vi "swabian_check_sync.vi"(8 "error in (no error)":errorcluster, 10 "Reference\nChannel":T1, 11 "swabian_local_data_IN":T2={"events"={"update_status"=refnum, "update_chart"=refnum, "update_xy"=refnum, "send_channel_data"=refnum}, "stop_q"=refnum, "tagger_reference"=refnum, "connect_button"=refnum, "counter_reference"=refnum, "tagger_stream_reference"=refnum, "log_reference"=refnum, "current_log_offset"=0, "tt20_buffer_q"=refnum, "stream_to_file_button"=refnum, "num_records"=0, "connected?"=FALSE, "plots"=refnum, "histogram_bin_edges"=[], "histogrammer"=refnum, "plot_lifetimes"=refnum, "xy_graph"=refnum, "Reference\nChannel"=enum."ch0", "trigger_channels"=[], "filter_channels"=[], "active_channels"=[], "acq_mode"=0, "Reference\nChannel"=enum."ch0", "acq_time"=0, "leftovers"={"leftover_stamps"=[], "leftover_channels"=[], "any?"=FALSE}, "sync_period_ps"=0, "raw_stream_path"=path "", "Leftovers"={"missing_sync_data"=[], "missing_events"=0}, "first_batch"=0, "first_sync_stamp"=0, "lifetime_settings"={"Plot Lifetimes"=FALSE, "start_time"=0.0, "stop_time"=0.0, "n_bins"=0}, "Histogram_bins"=[], "last_processed_data"=[], "histogram_data"=[]}) -> (0 "error out":errorcluster, 2 "sync_rate_hz":dbl, 3 "swabian_local_data":T2={"events"={"update_status"=refnum, "update_chart"=refnum, "update_xy"=refnum, "send_channel_data"=refnum}, "stop_q"=refnum, "tagger_reference"=refnum, "connect_button"=refnum, "counter_reference"=refnum, "tagger_stream_reference"=refnum, "log_reference"=refnum, "current_log_offset"=0, "tt20_buffer_q"=refnum, "stream_to_file_button"=refnum, "num_records"=0, "connected?"=FALSE, "plots"=refnum, "histogram_bin_edges"=[], "histogrammer"=refnum, "plot_lifetimes"=refnum, "xy_graph"=refnum, "Reference\nChannel"=enum."ch0", "trigger_channels"=[], "filter_channels"=[], "active_channels"=[], "acq_mode"=0, "Reference\nChannel"=enum."ch0", "acq_time"=0, "leftovers"={"leftover_stamps"=[], "leftover_channels"=[], "any?"=FALSE}, "sync_period_ps"=0, "raw_stream_path"=path "", "Leftovers"={"missing_sync_data"=[], "missing_events"=0}, "first_batch"=0, "first_sync_stamp"=0, "lifetime_settings"={"Plot Lifetimes"=FALSE, "start_time"=0.0, "stop_time"=0.0, "n_bins"=0}, "Histogram_bins"=[], "last_processed_data"=[], "histogram_data"=[]})   [LabVIEW 2018]
uses:
  swabian_local_data_tdef.ctl
  swabian_events_tdef.ctl
  update_chart_tdef.ctl
  channel_data_tdef.ctl
  C:/Users/bspoka/Documents/swabian_LV/lib/TTCSharp32.dll
  lib/TTCSharp32.dll
  swabian_buffer_tdef.ctl
  reference_checkbox_tdef.ctl
  leftovers_struct.ctl
  lifetime_settings.ctl
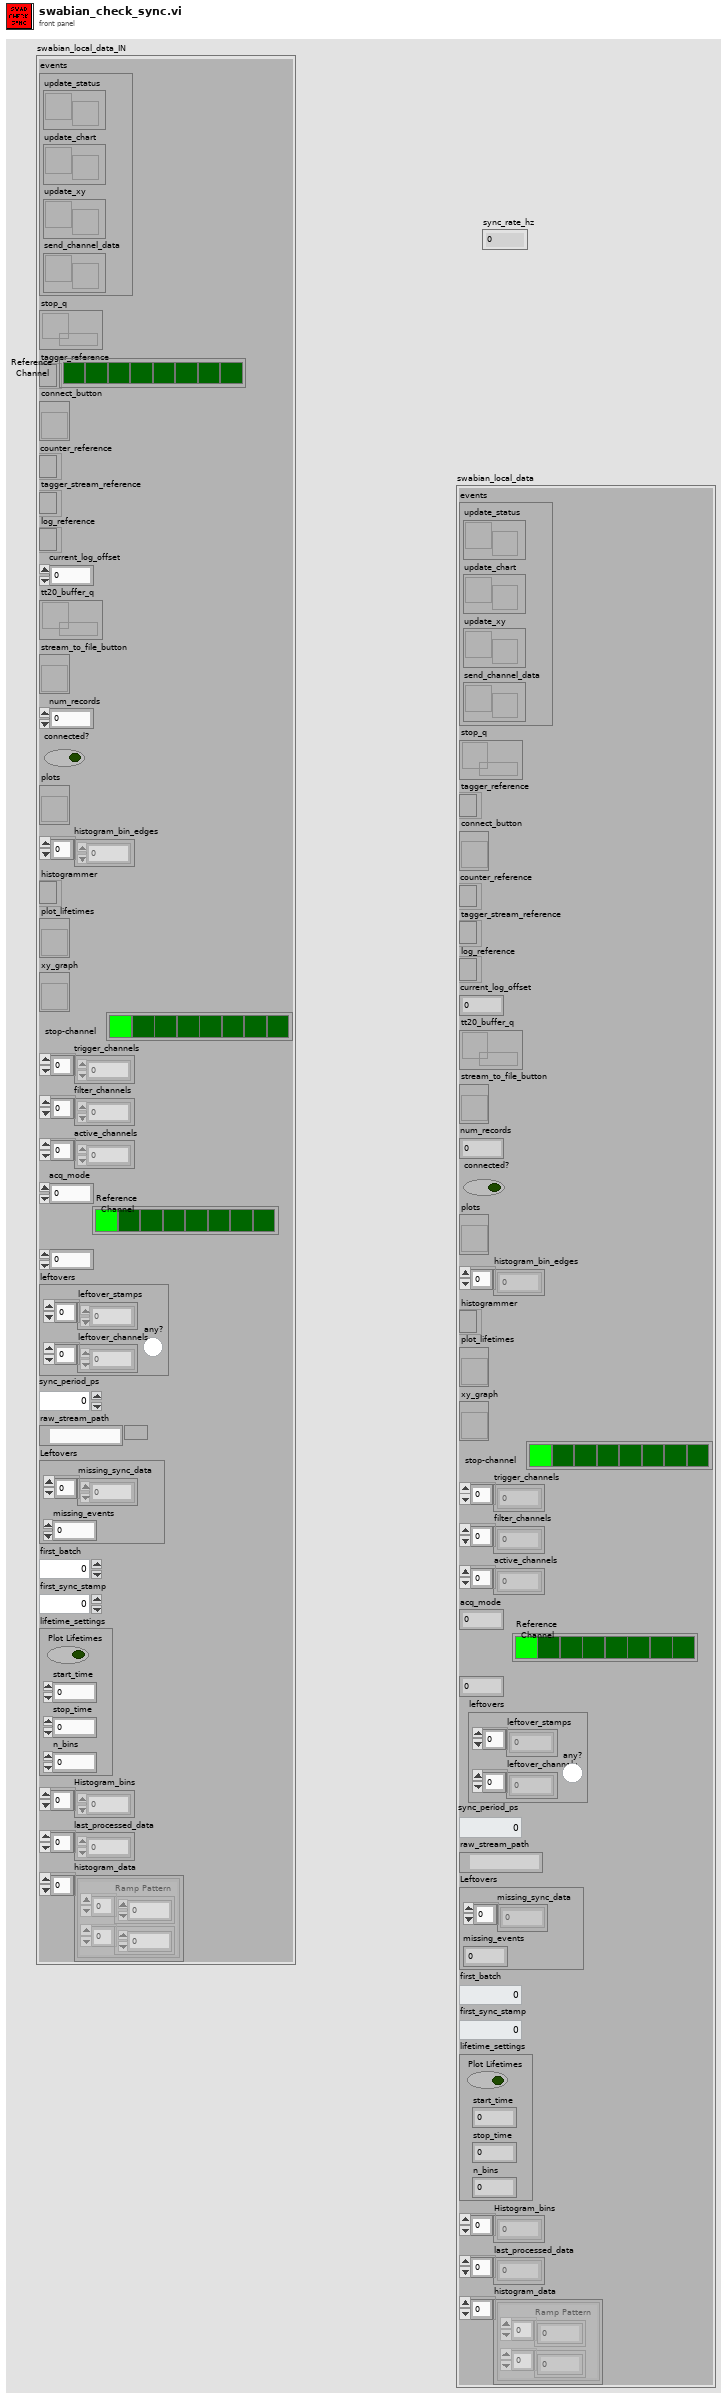
[diagram p1: front panel]
types:
  T1 = typedef "reference_checkbox_tdef.ctl" = enum32{"No Selection", "ch0", "ch1", "ch2", "ch3", "ch4", "ch5", "ch6", "ch7"}
  T2 = typedef "swabian_local_data_tdef.ctl" = cluster{"events":T3, "stop_q":refnum<queue>, "tagger_reference":refnum<k24>, "connect_button":refnum<vi>, "counter_reference":refnum<k24>, "tagger_stream_reference":refnum<k24>, "log_reference":refnum<file>, "current_log_offset":i64, "tt20_buffer_q":refnum<queue>, "stream_to_file_button":refnum<vi>, "num_records":u64, "connected?":bool, "plots":refnum<vi>, "histogram_bin_edges":i64[], "histogrammer":refnum<k24>, "plot_lifetimes":refnum<vi>, "xy_graph":refnum<vi>, "Reference\nChannel":T1, "trigger_channels":i32[], "filter_channels":i32[], "active_channels":i32[], "acq_mode":i32, "Reference\nChannel":T1, "acq_time":i64, "leftovers":T4, "sync_period_ps":i64, "raw_stream_path":path, "Leftovers":cluster{"missing_sync_data":u64[], "missing_events":i32}, "first_batch":i32, "first_sync_stamp":u64, "lifetime_settings":T5, "Histogram_bins":dbl[], "last_processed_data":u64[], "histogram_data":cluster{"Ramp Pattern":dbl[], dbl[]}[]}
  T3 = typedef "swabian_events_tdef.ctl" = cluster{"update_status":refnum<user-event>, "update_chart":refnum<user-event>, "update_xy":refnum<user-event>, "send_channel_data":refnum<user-event>}
  T4 = typedef "leftovers_struct.ctl" = cluster{"leftover_stamps":i64[], "leftover_channels":i32[], "any?":bool}
  T5 = typedef "lifetime_settings.ctl" = cluster{"Plot Lifetimes":bool, "start_time":dbl, "stop_time":dbl, "n_bins":i32}
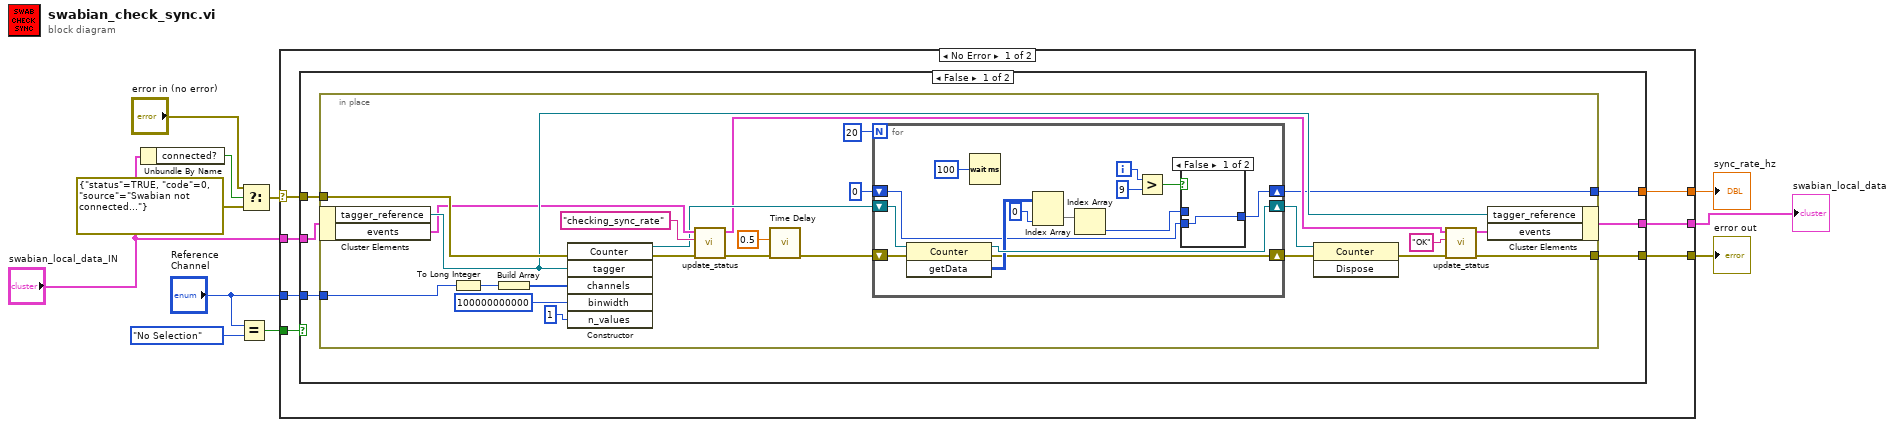
[diagram p0: block diagram]
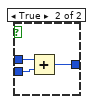
[diagram p2: hidden frame]
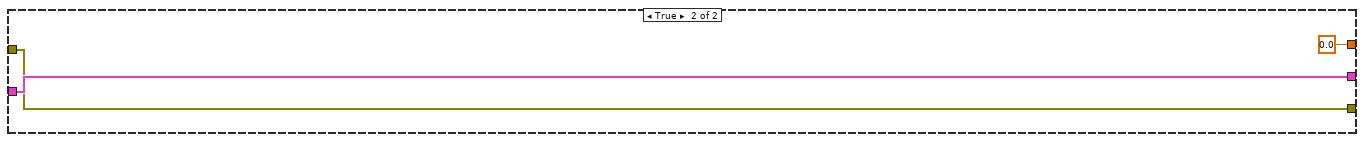
[diagram p3: hidden frame]
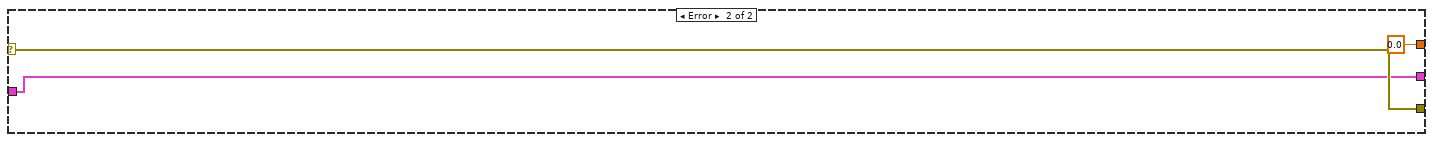
[diagram p4: hidden frame]
diagram:
  n1 = Unbundle By Name("swabian_local_data_IN") -> ("connected?"=w9:bool)
  n2 = Equal?(x="Reference\nChannel", y=reference_checkbox_tdef."No Selection") -> (x = y?=w3:bool)
  n3 = Select(t="error in (no error)", s=w9, f=errorcluster {"status"=TRUE, "code"=0, "source"="Swabian not connected..."}) -> (s? t:f=w5:errorcluster)
  n4 = case shown="No Error" w5 {
    selector: w5 -> [w17 w72]
    tunnel: "swabian_local_data_IN" -> [w18 w71]
    tunnel: [w16 w72] -> w11
    tunnel: [w15 w71] -> w10
    tunnel: w3 -> [w14 _]
    tunnel: "Reference\nChannel" -> [w13 _]
    tunnel: [w12 0.0] -> w1
    frame No Error {
      n5 = case shown="False" w14 {
        tunnel: w18 -> [w24 w69]
        tunnel: w17 -> [w23 w68]
        tunnel: [w22 w68] -> w16
        tunnel: [w21 w69] -> w15
        tunnel: w13 -> [w20 _]
        tunnel: [w19 0.0] -> w12
        frame False {
          n6 = in-place {
            in-place-border: w23 -> [w46]
            in-place-border: [w29] -> w22
            in-place-border: w20 -> [w40]
            in-place-border: [w25] -> w19
            n7 = in-place-cluster #1(w24) -> ("tagger_reference"=w45:refnum<k24>, "events"=w43:T3)
            n8 = To Long Integer(number=w40) -> (32bit integer=w39:i32)
            n9 = Build Array(w39) -> (w41:i32[])
            n10 = constructor class="Counter"(error in=w46, "tagger"=w45, "channels"=w41, "binwidth"=i64 100000000000, "n_values"=1) -> (reference out=w37:refnum<k24>, error out=w44:errorcluster)  [unwired: 2 in, 5 out]
            n11 = call "update_status.vi"("error in (no error)"=w44, "status"="checking_sync_rate", "events"=w43) -> ("error out"=w35:errorcluster, "events_out"=w28:T3)  [unwired: 7 in]
            n12 = call "Time Delay"("error in (no error)"=w35, "Delay Time (s)"=0.5) -> ("error out"=w34:errorcluster)  [unwired: 9 in]
            n13 = for {
              N: 20 -> [_]
              shift-right: [w52] -> w31
              shift-left: w34 -> [w60]
              shift-right: [w59] -> w32
              shift-left: w37 -> [w61]
              shift-right: [w55] -> w25
              shift-left: 0 ("element") -> [w53]
              i -> [w51]
              n14 = invoke class="Counter" method="getData"(reference=w61, error in=w60) -> (reference out=w59:refnum<k24>, error out=w52:errorcluster, "getData"=w58:i32[][])  [unwired: 1 in]
              n15 = Wait (ms)(milliseconds to wait=u32 100) -> ()  [unwired: 1 out]
              n16 = Index Array(array=w58, index (col)=0 ("index (row)")) -> (element=w56:i32[])  [unwired: 1 in]
              n17 = Index Array(array=w56) -> (element=w54:i32)  [unwired: 1 in]
              n18 = Greater?(x=w51, y=9) -> (0:w49:bool)
              n19 = case shown="False" w49 {
                tunnel: [w63 w66] -> w55
                tunnel: w54 -> [_ w65]
                tunnel: w53 -> [w63 w64]
                frame False {
                }
                frame True {
                  n20 = Add(x=w65, y=w64) -> (x+y=w66:i32)
                }
              }
            }
            n21 = invoke class="Counter" method="Dispose"(reference=w32, error in=w31) -> (error out=w30:errorcluster)  [unwired: 1 in, 2 out]
            n22 = call "update_status.vi"("error in (no error)"=w30, "status"="OK", "events"=w28) -> ("error out"=w29:errorcluster, "events_out"=w27:T3)  [unwired: 7 in]
            n23 = in-place-cluster #1("tagger_reference"=w45, "events"=w27) -> (w21:T2)
          }
        }
        frame True {
        }
      }
    }
    frame Error {
    }
  }
  "error out" <- w11
  "swabian_local_data" <- w10
  "sync_rate_hz" <- w1
